vi "GET Number of Samples [Slope Calibration].vi"() -> (0 "Number of Samples":dbl)   [LabVIEW 2013]
uses:
  Action.ctl
  Slope Calibration Inputs FGV Selector.ctl
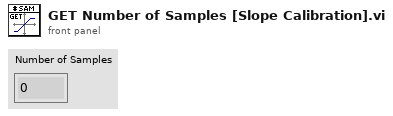
[diagram p1: front panel]
types:
  T1 = typedef "Slope Calibration Inputs FGV Selector.ctl" = enum16{"Number of Samples", "Ramp Rate", "Z Scan Size"}
  T2 = typedef "Action.ctl" = enum16{"GET", "PUT", "DELETE"}
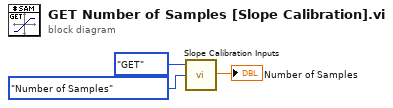
[diagram p0: block diagram]
diagram:
  n1 = call "Slope Calibration Inputs.vi"("Slope Calibration Inputs FGV Selector"=Slope_Calibration_Inputs_FGV_Selector."Number of Samples", "Action"=Action."GET") -> ("Output"=→"Number of Samples":dbl)  [unwired: 1 in]
